vi "to engine group.vi"(8 "Index":i32, 9 "Modbus Type":T2, 10 "Access":T8(ring), 11 "Channels":T1[](array[typedef])) -> (3 "Group":T7 {"VS Refs" format="%.0x"})   [LabVIEW 2015, in "Modbus Master System Explorer.lvlib"]
uses:
  Modbus Master System Explorer.lvlib
  Modbus Type.ctl
  <vilib>/NI Veristand/Custom Device API/Custom Device Item Ref.ctl
  Shared/Controls/Data Model/Channel.ctl
  <vilib>/NI Veristand/Custom Device API/Custom Device Channel Type.ctl
  Shared/Controls/Data Model/Mapping.ctl
  Shared/Controls/Data Model/DataType.ctl
  <vilib>/NI VeriStand/Custom Device API/Custom Device API.lvlib
  Shared/Modbus Master Shared.lvlib
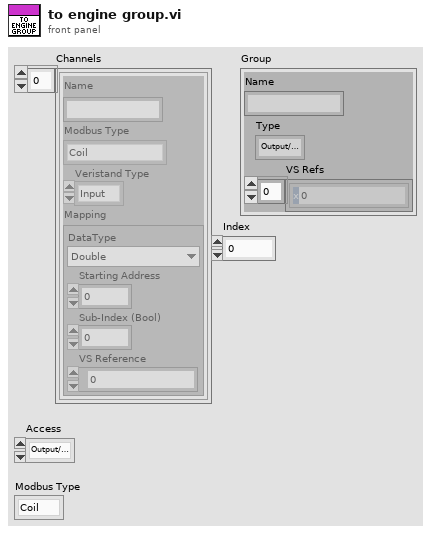
[diagram p1: front panel]
types:
  T1 = typedef "Modbus Master Shared.lvlib/Channel.ctl" = cluster{"Name":string, "Modbus Type":T2, "Veristand Type":T3, "Mapping":T4}
  T2 = typedef "Modbus Master Shared.lvlib/Modbus Type.ctl" = enum16{"Coil", "Discrete Input", "Holding Register", "Input Register"}
  T3 = typedef "Custom Device API.lvlib/Custom Device Channel Type.ctl" = enum16{"Input", "Output"}
  T4 = typedef "Modbus Master Shared.lvlib/Mapping.ctl" = cluster{"DataType":T5, "Starting Address":u16, "Sub-Index (Bool)":u16, "VS Reference":T6}
  T5 = typedef "Modbus Master Shared.lvlib/DataType.ctl" = enum16{"Double", "Single", "I64", "I32", "I16", "I8", "U64", "U32", "U16", "U8", "Boolean"}
  T6 = typedef "Custom Device API.lvlib/Custom Device Item Ref.ctl" = u64
  T7 = cluster{"Name":string, "Type":enum16{"Output/Write", "Input/Read", "Input/ReadWrite"}, "VS Refs":T6[]}
  T8 = enum16{"Output/Write", "Input/Read", "Input/ReadWrite"}
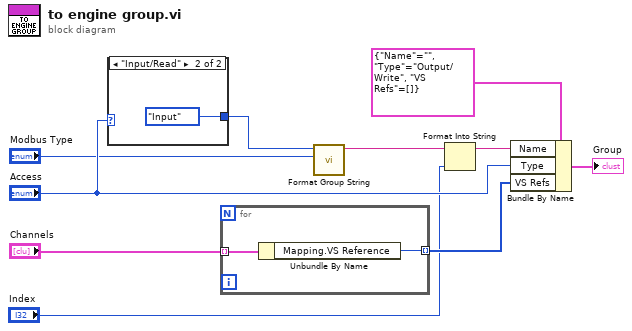
[diagram p0: block diagram]
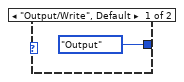
[diagram p2: hidden frame]
diagram:
  n1 = case shown="\"Input/Read\"" "Access" {
    tunnel: [Custom_Device_Channel_Type."Output" ("VS Type") Custom_Device_Channel_Type."Input" ("VS Type")] -> w7
    frame "Output/Write", Default {
    }
    frame "Input/Read" {
    }
  }
  n2 = for {
    tunnel: "Channels" -> [w14] mode=indexing
    tunnel: [w13] -> w4 mode=indexing
    n3 = Unbundle By Name(w14) -> ("Mapping.VS Reference"=w13:T6)
  }
  n4 = call "Format Group String.vi"("Modbus Type"="Modbus Type", "VS Type"=w7) -> ("Group String"=w2:string)  [unwired: 8 in, 1 out]
  n5 = Format Into String(initial string=w2, "Index") -> (resulting string=w1:string)  [unwired: 2 in, 1 out]
  n6 = Bundle By Name(cluster=T7 {"Name"="", "Type"=enum."Output/Write", "VS Refs"=[]} ("Group"), "Name"=w1, "Type"="Access", "VS Refs"=w4) -> (→"Group":T7)
